vi "AlliGator ucno_objective function phasor calibration.vi"(3 "output control":T1, 4 "data":variant, 5 "X":dbl[](array[numeric])) -> (0 "error out":errorcluster, 1 "gradient":dbl[](array[numeric]), 2 "f(X)":dbl)   [LabVIEW 2021, in "AlliGator Phasor Calibration.lvlib"]
doc: "Minimization function used to search for the optimal calibration based on two references."
uses:
  AlliGator Phasor Calibration.lvlib
  Variant/Variant to Data/Variant to [DBL].vi
  Variant/Variant to Data/Variant to Data.lvlib
panel:
  # "see the AlliGator License on the block diagram (Ctrl+E or Window:Show Block Diagram)"
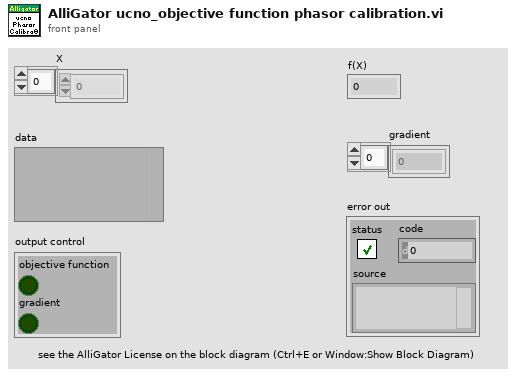
[diagram p1: front panel]
types:
  T1 = cluster{"objective function":bool, "gradient":bool}
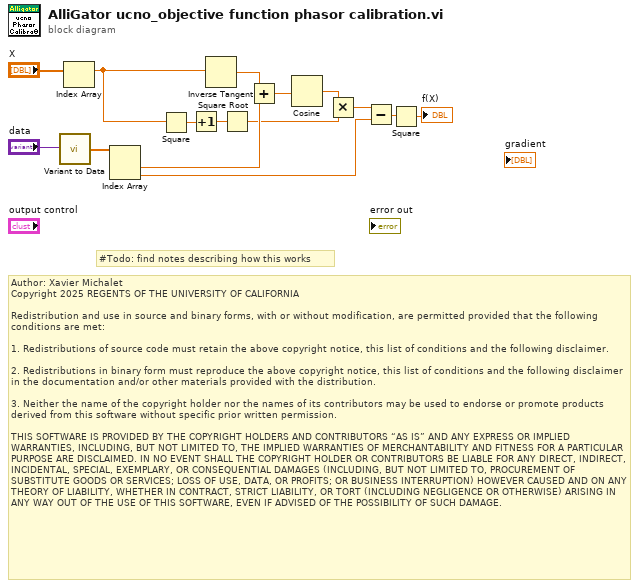
[diagram p0: block diagram]
diagram:
  # "Author: Xavier Michalet\nCopyright 2025 REGENTS OF THE UNIVERSITY OF CALIFORNIA\n\nRedistribution and use in source and binary forms, with or without modification, are permitted provided that the following conditions are met:\n\n1. Redistributions of source code must retain the above copyright notice, this list of conditions and the following disclaimer.\n\n2. Redistributions in binary form must reproduce the above copyright notice, this list of conditions and the following disclaimer in the documentation and/or other materials provided with the distribution.\n\n3. Neither the name of the copyright holder nor the names of its contributors may be used to endorse or promote products derived from this software without specific prior written permission.\n\nTHIS SOFTWARE IS PROVIDED BY THE COPYRIGHT HOLDERS AND CONTRIBUTORS “AS IS” AND ANY EXPRESS OR IMPLIED WARRANTIES, INCLUDING, BUT NOT LIMITED TO, THE IMPLIED WARRANTIES OF MERCHANTABILITY AND FITNESS FOR A PARTICULAR PURPOSE ARE DISCLAIMED. IN NO EVENT SHALL THE COPYRIGHT HOLDER OR CONTRIBUTORS BE LIABLE FOR ANY DIRECT, INDIRECT, INCIDENTAL, SPECIAL, EXEMPLARY, OR CONSEQUENTIAL DAMAGES (INCLUDING, BUT NOT LIMITED TO, PROCUREMENT OF SUBSTITUTE GOODS OR SERVICES; LOSS OF USE, DATA, OR PROFITS; OR BUSINESS INTERRUPTION) HOWEVER CAUSED AND ON ANY THEORY OF LIABILITY, WHETHER IN CONTRACT, STRICT LIABILITY, OR TORT (INCLUDING NEGLIGENCE OR OTHERWISE) ARISING IN ANY WAY OUT OF THE USE OF THIS SOFTWARE, EVEN IF ADVISED OF THE POSSIBILITY OF SUCH DAMAGE."
  # "#Todo: find notes describing how this works"
  n1 = call-poly "Variant to Data.vi"("Variant"="data") -> ("Value"=w14:dbl[])  [unwired: 8 in]
  n2 = Index Array(array="X") -> (element=w2:dbl)  [unwired: 1 in]
  n3 = Index Array(array=w14) -> (element #1=w12:dbl, element #2=w4:dbl)  [unwired: 2 in]
  n4 = Square(x=w2) -> (x^2=w9:dbl)
  n5 = Increment(x=w9) -> (x+1=w8:dbl)
  n6 = Inverse Tangent(1:w2) -> (0:w13:dbl)
  n7 = Square Root(x=w8) -> (sqrt(x)=w6:dbl)
  n8 = Add(x=w13, y=w12) -> (x+y=w11:dbl)
  n9 = Cosine(x=w11) -> (cos(x)=w7:dbl)
  n10 = Multiply(x=w7, y=w6) -> (x*y=w5:dbl)
  n11 = Subtract(x=w5, y=w4) -> (x-y=w3:dbl)
  n12 = Square(x=w3) -> (x^2=→"f(X)":dbl)
